vi "Write Multiple Input Registers.vi"(8 "error in":errorcluster, 9 "input registers to write":u16[](array[numeric]), 10 "starting address":u16, 11 "Modbus slave in":refnum<class "Modbus Slave.lvclass">) -> (0 "error out":errorcluster, 3 "Modbus slave out":refnum<class "Modbus Slave.lvclass">)   [LabVIEW 2015, in "Modbus Library.lvlib" / "Modbus Slave.lvclass"]
doc: "Writes <B>input registers to write</B> starting at <B>starting address</B> to the device registers. This function is usable by the Modbus slave only."
uses:
  Modbus Slave.lvclass
  Modbus Slave.lvclass/Modbus Slave.ctl
  Data Model/Device Data Model.lvclass
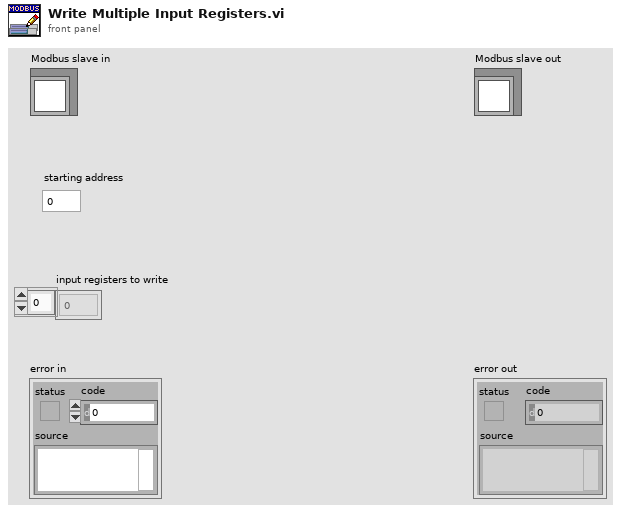
[diagram p1: front panel]
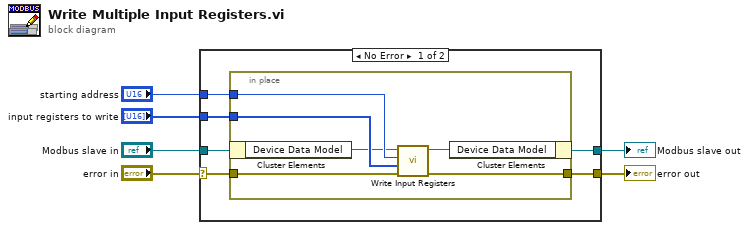
[diagram p0: block diagram]
diagram:
  n1 = case shown="No Error" "error in" {
    selector: "error in" -> [w10 w20]
    tunnel: [w7 w20] -> w4
    tunnel: "Modbus slave in" -> [w8 w19]
    tunnel: "input registers to write" -> [w12 _]
    tunnel: "starting address" -> [w11 _]
    tunnel: [w9 w19] -> w1
    frame No Error {
      n2 = in-place {
        in-place-border: w12 -> [w18]
        in-place-border: w11 -> [w17]
        in-place-border: w10 -> [w16]
        in-place-border: [w15] -> w7
        n3 = in-place-cluster #1(w8) -> ("Device Data Model"=w13:refnum<class "Device Data Model.lvclass">)
        n4 = call-dynamic "Write Input Registers.vi"("error in (no error)"=w16, "register values"=w18, "starting address"=w17, "Device Data Model in"=w13) -> ("error out"=w15:errorcluster, "Device Data Model out"=w14:refnum<class "Device Data Model.lvclass">)  [unwired: 6 in]
        n5 = in-place-cluster #1("Device Data Model"=w14) -> (w9:refnum<class "Modbus Slave.lvclass">)
      }
    }
    frame Error {
    }
  }
  "error out" <- w4
  "Modbus slave out" <- w1
